vi "Test VI.vi"() -> ()   [LabVIEW 2019, in "Test Class.lvclass"]
uses:
  Test Class.lvclass
panel:
  in  "Path":path
  in  "String":string
  in  "Listbox":i32(listbox)
  out "Time Stamp":timestamp
  out "Slide 3":u8(slide) scale=0.0..100.0
  in  "Knob":dbl(knob) scale=0.0..10.0
  in  "Slide 2":dbl(slide) scale=0.0..10.0
  in  "Slide":dbl(slide) scale=0.0..10.0
  in  "Numeric":dbl
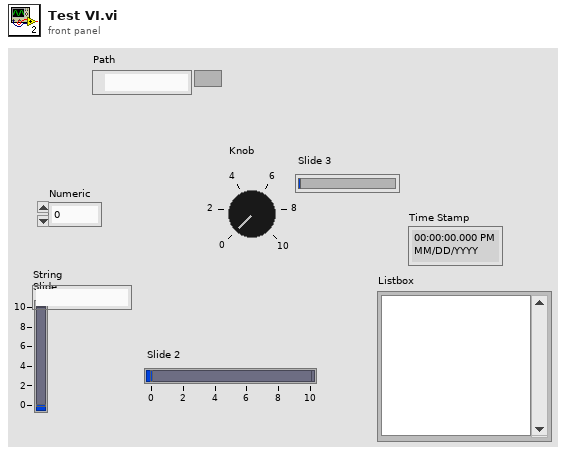
[diagram p1: front panel]
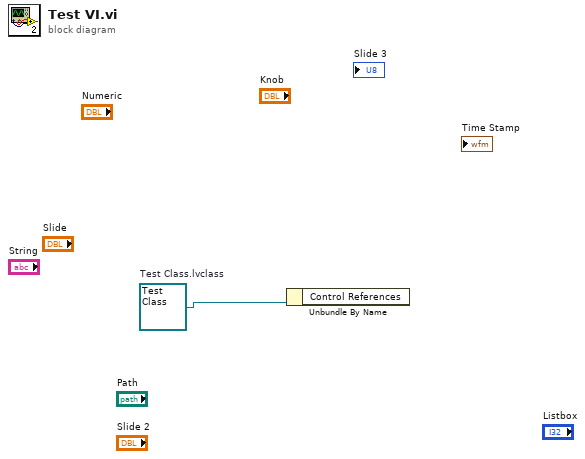
[diagram p0: block diagram]
diagram:
  w1 = refnum<class "Test Class.lvclass"> refnum  # Test Class.lvclass
  n1 = Unbundle By Name(w1) -> ()  [unwired: 1 out]
